vi "Main.vi"() -> ()   [LabVIEW 2020, in "Amnesia.lvlib"]
uses:
  Amnesia.lvlib
  Scene/Scene.lvclass/Scene.ctl
  Scene/Mouse Button Held.ctl
  Scene/Scene.lvclass
  <vilib>/Dataflow_G/G-Audio/G-Audio.lvlib
panel:
  out "Screen":picture
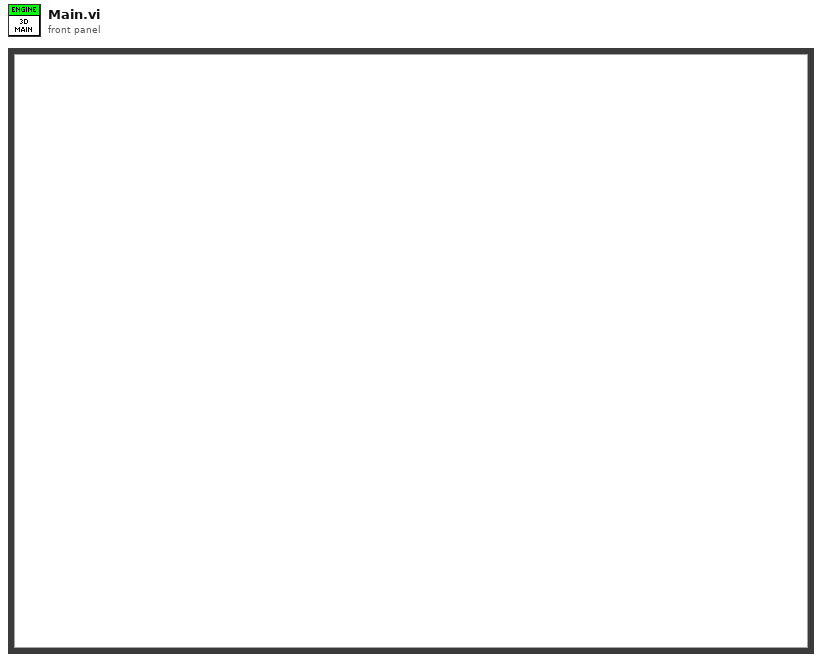
[diagram p1: front panel]
types:
  T1 = typedef "Amnesia.lvlib/Core Data.ctl" = cluster{"Pixel Data":u32[][], "Scene":refnum<class "Scene.lvclass">, "Mouse Button Held":T2, "Audio Device":T3}
  T2 = typedef "Scene.lvclass/Mouse Button Held.ctl" = enum16{"None", "Left", "Middle", "Right"}
  T3 = typedef "G-Audio.lvlib/Audio Device Refnum.ctl" = refnum<file>
  T4 = enum32{"invalid app kind", "Development System", "Run Time System", "Student Edition", "Embedded LabVIEW", "Evaluation", "Custom"}
  T5 = typedef "LVPoint32TypeDef.ctl" = cluster{"Horizontal":i32, "Vertical":i32}
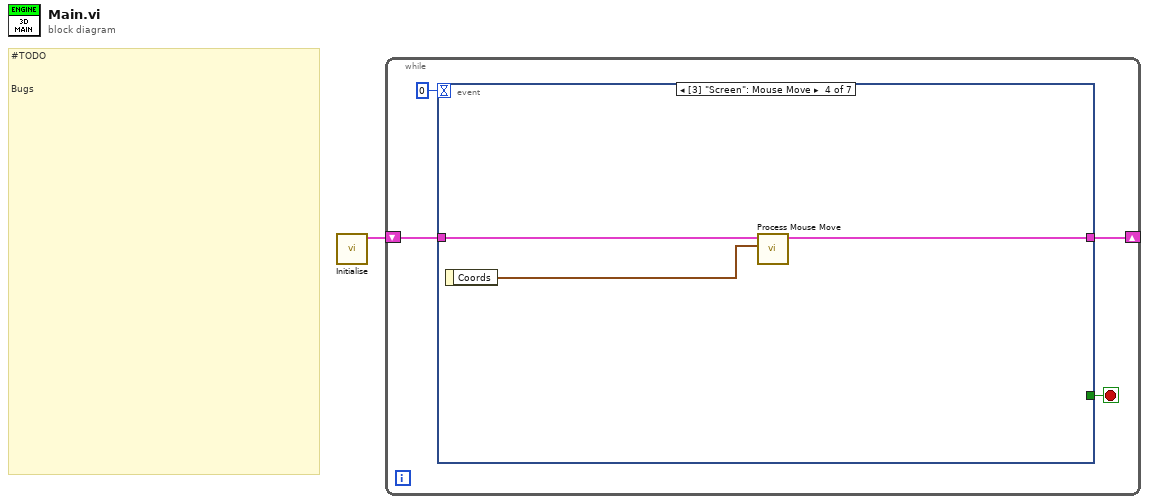
[diagram p0: block diagram]
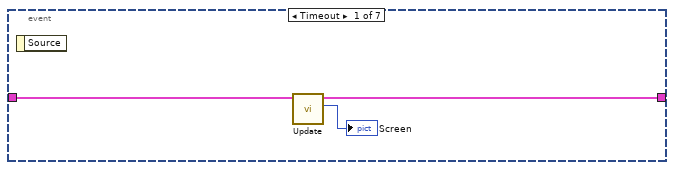
[diagram p2: hidden frame]
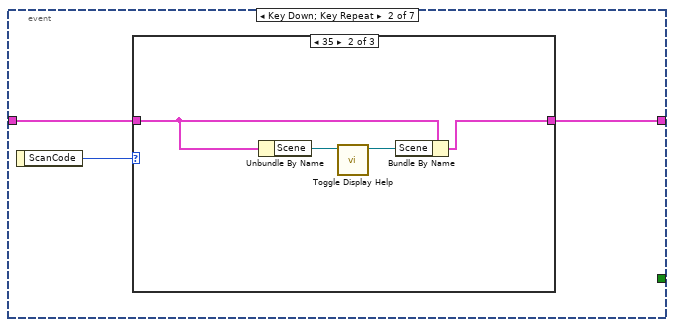
[diagram p3: hidden frame]
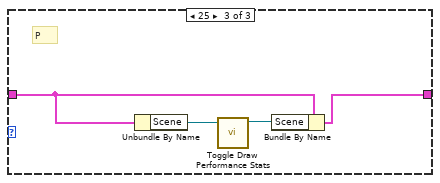
[diagram p5: hidden frame]
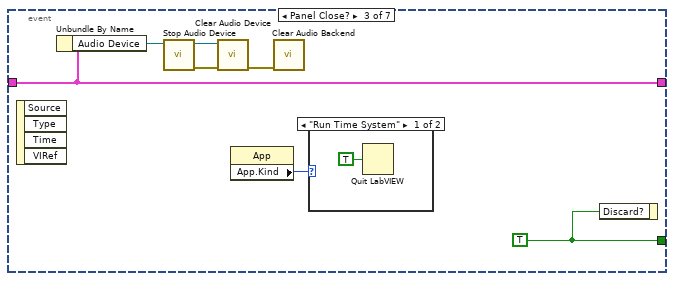
[diagram p6: hidden frame]
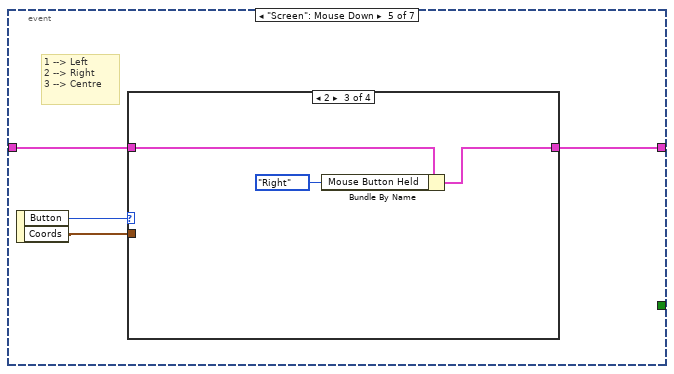
[diagram p8: hidden frame]
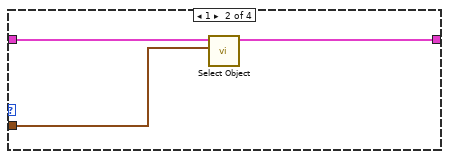
[diagram p10: hidden frame]
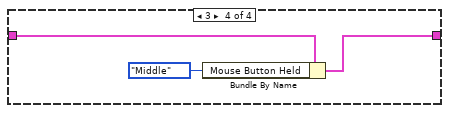
[diagram p11: hidden frame]
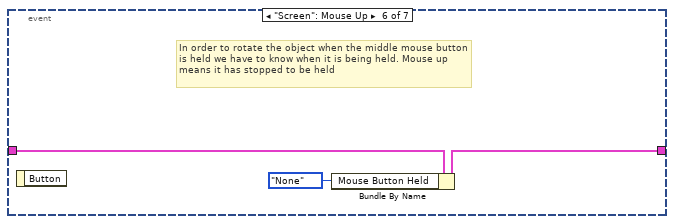
[diagram p12: hidden frame]
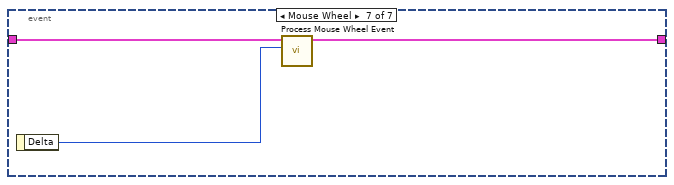
[diagram p13: hidden frame]
diagram:
  # "#TODO\n\n\nBugs"
  n1 = call "Initialise.vi"() -> ("Core Data out"=w1:T1)  [unwired: 11 in]
  n2 = while {
    shift-right: [w4] -> _
    shift-left: w1 -> [w5]
    stop <- w3 stop-if-true
    n3 = event shown="[3] \"Screen\": Mouse Move" {
      selector: _ -> [_ _ _ _ _ _ _]
      dyn-events: _ -> [_ _ _ _ _ _ _]
      timeout: 0 -> [_ _ _ _ _ _ _]
      tunnel: w5 -> [w6 w10 w25 w30 w34 w48 w50]
      tunnel: [w8 w9 w25 w31 w33 w47 w51] -> w4
      tunnel: [_ _ w27 _ _ _ _] -> w3
      event Timeout {
        n4 = event-data() -> ()  [unwired: 1 in, 1 out]
        n5 = call "Update.vi"("Core Data in"=w6) -> ("Screen"=→"Screen":picture, "Core Data out"=w8:T1)  [unwired: 9 in]
      }
      event Key Down; Key Repeat {
        n6 = event-data() -> ("ScanCode"=w11:i16)  [unwired: 1 in]
        n7 = case shown="35" w11 {
          tunnel: w10 -> [w12 w14 w20]
          tunnel: [w12 w13 w19] -> w9
          frame Default {
          }
          frame 35 {
            n8 = Unbundle By Name(w14) -> ("Scene"=w15:refnum<class "Scene.lvclass">)
            n9 = call "Toggle Display Help.vi"("Scene in"=w15) -> ("Scene out"=w16:refnum<class "Scene.lvclass">)  [unwired: 10 in]
            n10 = Bundle By Name(cluster=w14, "Scene"=w16) -> (w13:T1)
          }
          frame 25 {
            # "P"
            n11 = Unbundle By Name(w20) -> ("Scene"=w18:refnum<class "Scene.lvclass">)
            n12 = call "Toggle Draw Performance Stats.vi"("Scene in"=w18) -> ("Scene out"=w17:refnum<class "Scene.lvclass">)  [unwired: 10 in]
            n13 = Bundle By Name(cluster=w20, "Scene"=w17) -> (w19:T1)
          }
        }
      }
      event Panel Close? {
        w27 = TRUE ("Discard?")
        (unwired) TRUE ("Discard?")
        n14 = event-data() -> ()  [unwired: 1 in, 4 out]
        n15 = Unbundle By Name(w25) -> ("Audio Device"=w21:T3)
        n16 = call <vilib>:"Stop Audio Device.vi"("Audio Device Refnum In"=w21) -> ("error out"=w23:errorcluster, "Audio Device Refnum Out"=w22:T3)  [unwired: 9 in]
        n17 = call <vilib>:"Clear Audio Device.vi"("error in (no error)"=w23, "Audio Device Refnum In"=w22) -> ("error out"=w24:errorcluster)  [unwired: 9 in]
        n18 = property class="App"() -> ("App.Kind"=w26:T4)  [unwired: 2 in, 2 out]
        n19 = call <vilib>:"Clear Audio Backend.vi"("error in (no error)"=w24) -> ()  [unwired: 10 in, 1 out]
        n20 = case shown="\"Run Time System\"" w26 {
          frame "Run Time System" {
            n21 = Quit LabVIEW(quit? (T)=TRUE) -> ()
          }
          frame Default {
          }
        }
        n22 = event-data("Discard?"=w27) -> ()  [unwired: 1 in, 1 out]
      }
      event "Screen": Mouse Move {
        n23 = event-data() -> ("Coords"=w29:T5)  [unwired: 1 in]
        n24 = call "Process Mouse Move.vi"("Coords"=w29, "Core Data in"=w30) -> ("Core Data out"=w31:T1)  [unwired: 9 in]
      }
      event "Screen": Mouse Down {
        # "1 --> Left\n2 --> Right\n3 --> Centre"
        n25 = event-data() -> ("Button"=w35:u16, "Coords"=w32:T5)  [unwired: 1 in]
        n26 = case shown="2" w35 {
          tunnel: w34 -> [w36 w39 w42 w45]
          tunnel: [w36 w38 w40 w43] -> w33
          tunnel: w32 -> [_ w37 _ _]
          frame Default {
          }
          frame 1 {
            n27 = call "Select Object.vi"("Coords"=w37, "Core Data in"=w39) -> ("Core Data out"=w38:T1)  [unwired: 8 in, 1 out]
          }
          frame 2 {
            n28 = Bundle By Name(cluster=w42, "Mouse Button Held"=Mouse_Button_Held."Right") -> (w40:T1)
          }
          frame 3 {
            n29 = Bundle By Name(cluster=w45, "Mouse Button Held"=Mouse_Button_Held."Middle") -> (w43:T1)
          }
        }
      }
      event "Screen": Mouse Up {
        # "In order to rotate the object when the middle mouse button is held we have to know when it is being held. Mouse up means it has stopped to be held"
        n30 = event-data() -> ()  [unwired: 1 in, 1 out]
        n31 = Bundle By Name(cluster=w48, "Mouse Button Held"=Mouse_Button_Held."None") -> (w47:T1)
      }
      event Mouse Wheel {
        n32 = event-data() -> ("Delta"=w49:i32)  [unwired: 1 in]
        n33 = call "Process Mouse Wheel Event.vi"("Delta"=w49, "Core Data in"=w50) -> ("Core Data out"=w51:T1)  [unwired: 9 in]
      }
    }
  }
